vi "Create Sessions.vi"   [LabVIEW 2020, in "Keysight 34401A DMM Instrument.lvlib"]
doc: "Create the 34401 driver session(s) from a reservation."
uses:
  Keysight 34401A DMM Instrument.lvlib
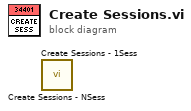
[diagram p0: block diagram]
diagram:
  n1 = call "Create Sessions - NSess.vi"() -> ()  [unwired: 8 in, 4 out]
  n2 = call "Create Sessions - 1Sess.vi"() -> ()  [unwired: 8 in, 4 out]
